vi "dIMU_Accel_ms.vi"(7 "Port":T1 items=["Port 1", "Port 2", "Port 3", "Port 4"], 8 "Calibrate":bool, 9 "Maximum Range":enum8{"2g", "4g", "8g"}(ring), 10 "Calibrate Axis":enum8{"Z", "X", "Y"}(ring), 11 "NXT":T2) -> (0 "Z Accel (m/s)":dbl, 1 "Y Accel (m/s)":dbl, 2 "X Accel (m/s)":dbl, 3 "NXT":T2)   [LabVIEW 2010]
uses:
  <vilib>/NXT/Subs/LVHSConnector.ctl
  <vilib>/NXT/Block Support/NXT_InputPort.ctl
  <vilib>/NXT/Block Support/HWPage.SensorType.ctl
  <vilib>/NXT/Block Support/HWPage.SensorMode.ctl
  <vilib>/NXT/Dual Mode Library/Sensors/i2c_sensors.vi
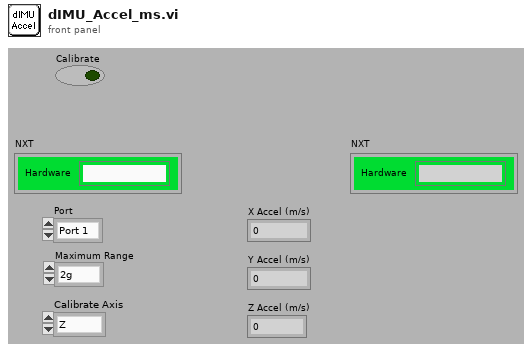
[diagram p1: front panel]
types:
  T1 = typedef "NXT_InputPort.ctl" = u8
  T2 = typedef "LVHSConnector.ctl" = cluster{"Hardware":string, "Flattened String":string}
  T3 = typedef "HWPage.SensorType.ctl" = u8
  T4 = typedef "HWPage.SensorMode.ctl" = u8
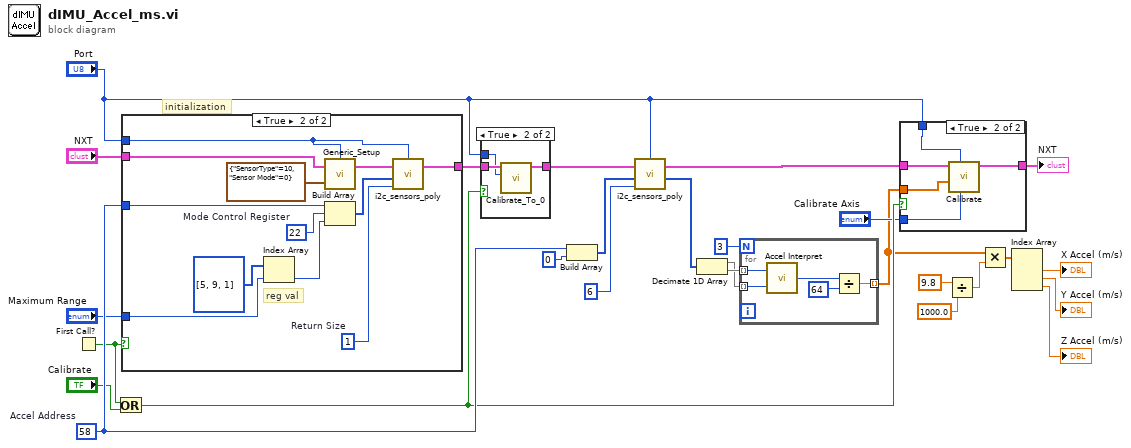
[diagram p0: block diagram]
diagram:
  w25 = u8 58  # Accel Address
  # "initialization"
  n1 = First Call?() -> (First Call?: T/F=w15:bool)
  n2 = Or(x=w15, y="Calibrate") -> (x .or. y?=w13:bool)
  n3 = case shown="True" w15 {
    tunnel: "Maximum Range" -> [_ w39]
    tunnel: "NXT" -> [w28 w38]
    tunnel: [w28 w32] -> w17
    tunnel: "Port" -> [_ w31]
    tunnel: w25 -> [_ w30]
    frame False {
    }
    frame True {
      w33 = u8 1  # Return Size
      w36 = u8 22  # Mode Control Register
      # "reg val"
      n4 = Index Array(array=u8[] [5, 9, 1], index=w39) -> (element=w35:u8)
      n5 = call <vilib>:"Generic_Setup.vi"("Sensor Setup"=cluster{"SensorType":T3, "Sensor Mode":T4} {"SensorType"=10, "Sensor Mode"=0}, "NXT"=w38, "Port"=w31) -> ("NXT"=w37:T2)  [unwired: 1 out]
      n6 = Build Array(w30, w36, w35) -> (w34:u8[])
      n7 = call-poly <vilib>:"i2c_sensors_poly.vi"("Return Length"=w33, "Bytes to Write"=w34, "NXT"=w37, "Port"=w31) -> ("NXT"=w32:T2)  [unwired: 1 in, 2 out]
    }
  }
  n8 = case shown="True" w13 {
    tunnel: w17 -> [w41 w44]
    tunnel: [w41 w43] -> w16
    tunnel: "Port" -> [_ w42]
    frame False {
    }
    frame True {
      n9 = call "Calibrate_To_0.vi"("Port"=w42, "NXT"=w44) -> ("NXT 2"=w43:T2)  [unwired: 9 in]
    }
  }
  n10 = Build Array(w25, u8 0) -> (w23:u8[])
  n11 = call-poly <vilib>:"i2c_sensors_poly.vi"("Return Length"=u8 6, "Bytes to Write"=w23, "NXT"=w16, "Port"="Port") -> ("Bytes read"=w22:u8[], "NXT"=w11:T2)  [unwired: 1 in, 1 out]
  n12 = Decimate 1D Array(w22) -> (w20:u8[], w21:u8[])
  n13 = for {
    N: 3 -> [_]
    tunnel: w21 -> [w49] mode=indexing
    tunnel: w20 -> [w48] mode=indexing
    tunnel: [w45] -> w4 mode=indexing
    n14 = call "Accel Interpret.vi"("LSB"=w48, "MSB"=w49) -> ("Value"=w46:i16)
    n15 = Divide(x=w46, y=i16 64) -> (x/y=w45:dbl)
  }
  n16 = case shown="True" w13 {
    tunnel: w11 -> [w50 w55]
    tunnel: "Port" -> [_ w51]
    tunnel: "Calibrate Axis" -> [_ w53]
    tunnel: w4 -> [_ w54]
    tunnel: [w50 w52] -> w10
    frame False {
    }
    frame True {
      n17 = call "Calibrate.vi"("Calibrate Axis"=w53, "Port"=w51, "Accel Input Array"=w54, "NXT"=w55) -> ("NXT"=w52:T2)  [unwired: 7 in]
    }
  }
  "NXT" <- w10
  n18 = Divide(x=9.8, y=1000.0) -> (x/y=w1:dbl)
  n19 = Multiply(x=w4, y=w1) -> (x*y=w5:dbl[])
  n20 = Index Array(array=w5) -> (element #1=→"X Accel (m/s)":dbl, element #2=→"Y Accel (m/s)":dbl, element #3=→"Z Accel (m/s)":dbl)  [unwired: 3 in]
